vi "Sub_GBD_FileConvert.vi"(8 "error in (no error)":errorcluster, 10 "CSV":path caption="出力パス", 11 "GBD":path caption="ファイル") -> (0 "error out":errorcluster, 1 "EOF":bool)   [LabVIEW 2017]
panel:
  in  "Cancel Button":bool
  out "Slide":dbl(slide) scale=0.0..1.0
  in  "Param":cluster{"START":i32, "End":i32, "Delta":i32}={"START"=0, "End"=-1, "Delta"=1}
  # "ファイル変換中..."
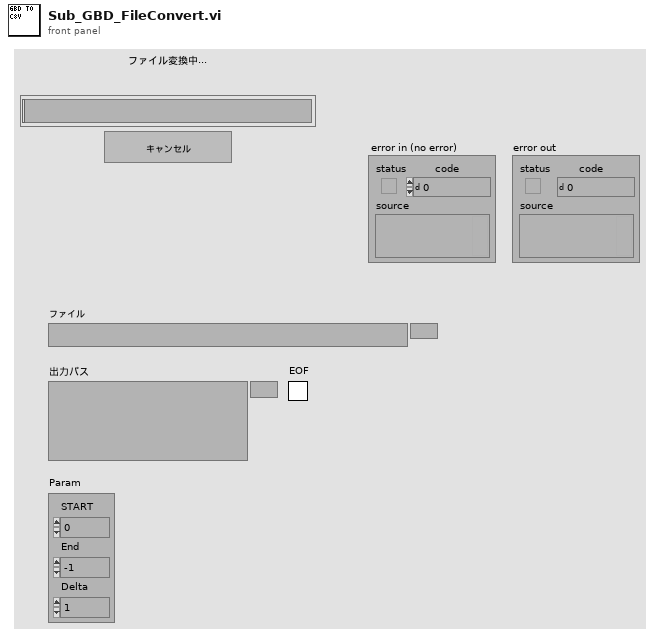
[diagram p1: front panel]
types:
  T1 = typedef "Amp_Param.ctl" = cluster{"File":refnum<file>[], "Idx":refnum<file>[], "dT":dbl, "Hd":i32, "Rd":i32, "Start":timestamp[], "Trig":timestamp[], "Stop":timestamp[], "FirstPos":timestamp[], "Count":i64[], "Color":u32[], "Label":string[], "INP":string[], "H":dbl[], "L":dbl[], "Fmt":string[], "Unit":string[], "SEL":i32[], "Byte":i32[], "Pos":i32[], "Bit":i32[], "Flg":i32[], "Gain":dbl[], "Offset":dbl[], "CH":i32[], "Opt":cluster{"Mode":i32, "TUNIT":enum16{"CELS", "FAHR"}}, "TYPE":enum16{"GBD", "CSV"}, "Comp":refnum<file>[], "Temp":i32[]}
  T2 = enum16{"open", "replace", "create", "open or create", "replace or create", "replace or create with confirmation"}
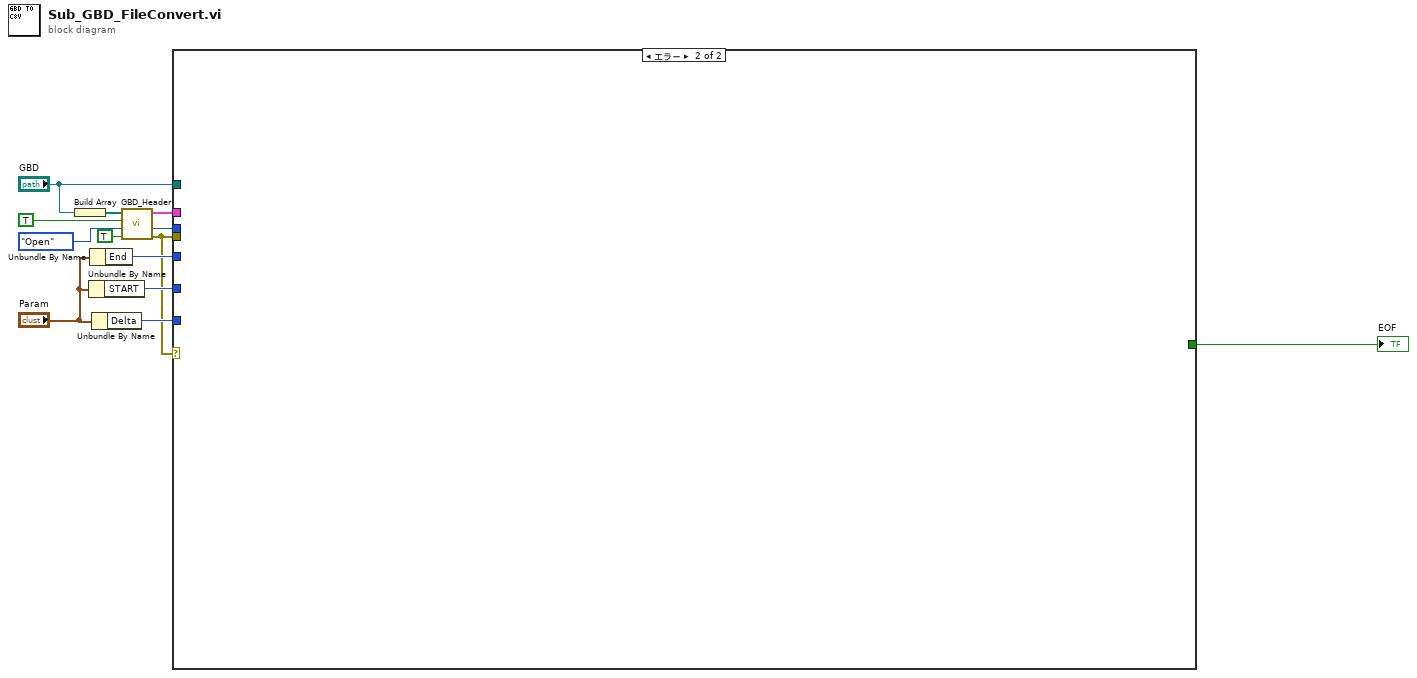
[diagram p0: block diagram]
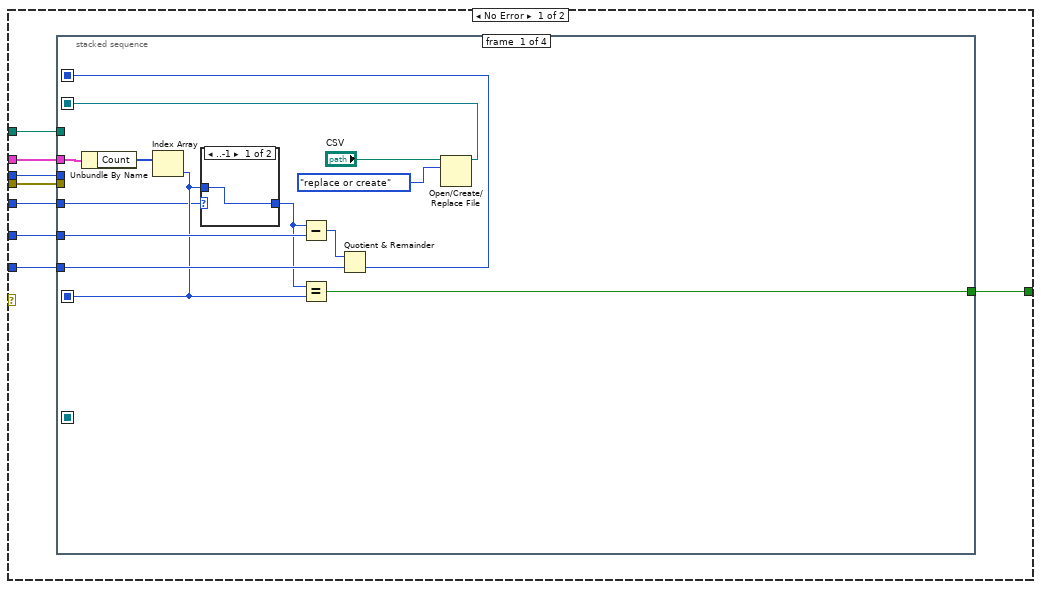
[diagram p2: hidden frame]
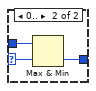
[diagram p3: hidden frame]
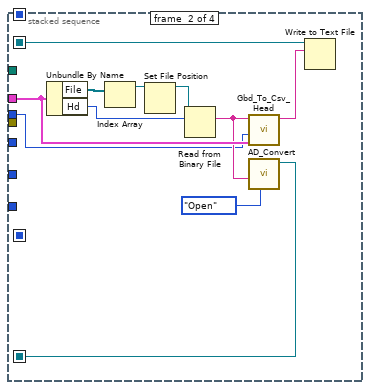
[diagram p4: hidden frame]
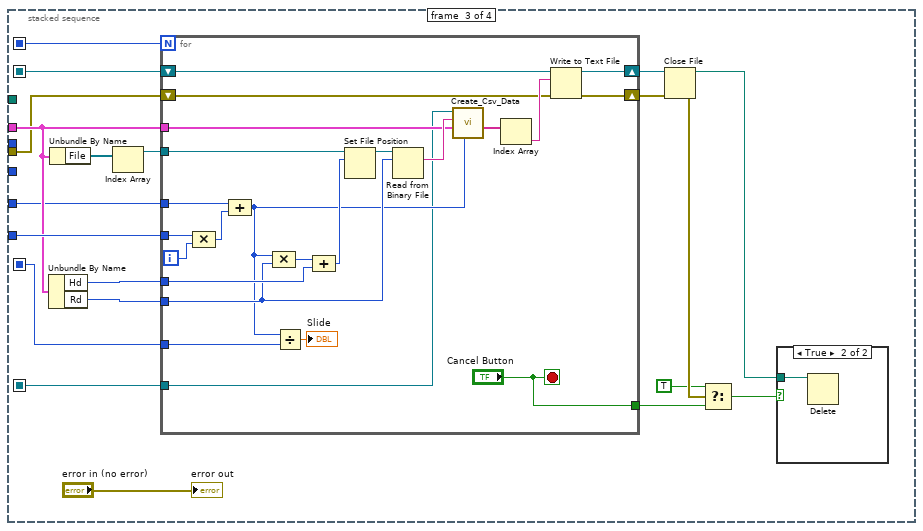
[diagram p5: hidden frame]
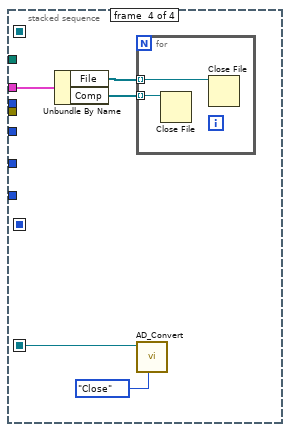
[diagram p7: hidden frame]
diagram:
  n1 = Build Array("GBD") -> (w3:path[])
  n2 = Unbundle By Name("Param") -> ("START"=w11:i32)
  n3 = Unbundle By Name("Param") -> ("End"=w12:i32)
  n4 = Unbundle By Name("Param") -> ("Delta"=w13:i32)
  n5 = call "GBD_Header.vi"("Save?"=TRUE, "Mode"=enum16{"Open", "Close", "Index"}."Open", "Cvt_Mode"=TRUE, "File[]"=w3) -> ("error out"=w1:errorcluster, "ActiveCH"=w2:i32, "Param"=w5:T1)  [unwired: 3 in, 2 out]
  n6 = case shown="エラー" w1 {
    tunnel: w13 -> [w21 _]
    tunnel: w12 -> [w20 _]
    tunnel: w11 -> [w19 _]
    tunnel: [w18 _] -> w9
    tunnel: "GBD" -> [w17 _]
    tunnel: w5 -> [w16 _]
    tunnel: w1 -> [w15 _]
    tunnel: w2 -> [w14 _]
    frame No Error {
      n7 = stacked-sequence {
        seq-local: [w33 _ _ _] -> [_ w45 w58 _]
        seq-local: [w28 _ _ _] -> [_ _ w64 _]
        seq-local: [w25 _ _ _] -> [_ _ w63 _]
        seq-local: [_ w40 _ _] -> [_ _ w55 w95]
        tunnel: w17 -> [_ _ _ _]
        tunnel: w19 -> [w31 _ w60 _]
        tunnel: w21 -> [w29 _ w65 _]
        tunnel: w20 -> [w24 _ _ _]
        tunnel: [w26 _ _ _] -> w18
        tunnel: w16 -> [w22 w43 w61 w98]
        tunnel: w15 -> [_ _ w54 _]
        tunnel: w14 -> [_ w39 _ _]
        frame #0 {
          n8 = Unbundle By Name(w22) -> ("Count"=w32:i64[])
          n9 = Index Array(array=w32) -> (element=w25:i64)  [unwired: 1 in]
          n10 = case shown="..-1" w24 {
            selector: w24 -> [_ w36]
            tunnel: [w35 w38] -> w27
            tunnel: w25 -> [w35 w37]
            frame ..-1 {
            }
            frame 0.. {
              n11 = Max & Min(x=w37, y=w36) -> (min(x,y)=w38:i64)  [unwired: 1 out]
            }
          }
          n12 = Subtract(x=w27, y=w31) -> (x-y=w30:i64)
          n13 = Equal?(x=w27, y=w25) -> (x = y?=w26:bool)
          n14 = Quotient & Remainder(x=w30, y=w29) -> (floor(x/y)=w28:i64)  [unwired: 1 out]
          n15 = Open/Create/Replace File(file path (use dialog)="CSV", operation (0:open)=T2."replace or create") -> (refnum out=w33:refnum<file>)  [unwired: 4 in, 2 out]
        }
        frame #1 {
          n16 = Unbundle By Name(w43) -> ("File"=w49:refnum<file>[], "Hd"=w46:i32)
          n17 = Index Array(array=w49) -> (element=w48:refnum<file>)  [unwired: 1 in]
          n18 = Set File Position(refnum=w48) -> (refnum out=w47:refnum<file>)  [unwired: 3 in, 1 out]
          n19 = Read from Binary File(10:w46, 11:w47) -> (2:w42:string)  [unwired: 4 in, 3 out]
          n20 = call "Gbd_To_Csv_Head.vi"("Param"=w43, "数値"=w39, "GBD"=w42) -> ("CSV"=w44:string)  [unwired: 8 in]
          n21 = call "AD_Convert.vi"("Mode"=enum16{"Open", "Convert", "Close"}."Open", "Header"=w42) -> ("Reference.Out"=w40:refnum<k24>)  [unwired: 7 in, 2 out]
          n22 = Write to Text File(file (use dialog)=w45, text=w44) -> ()  [unwired: 2 in, 3 out]
        }
        frame #2 {
          n23 = Unbundle By Name(w61) -> ("Hd"=w66:i32, "Rd"=w67:i32)
          n24 = Unbundle By Name(w61) -> ("File"=w69:refnum<file>[])
          n25 = Index Array(array=w69) -> (element=w68:refnum<file>)  [unwired: 1 in]
          n26 = for {
            N: w64 -> [_]
            tunnel: w68 -> [w93]
            tunnel: w67 -> [w87]
            tunnel: w66 -> [w90]
            tunnel: w60 -> [w83]
            tunnel: w65 -> [w85]
            tunnel: w63 -> [w81]
            tunnel: w61 -> [w78]
            tunnel: ["Cancel Button"] -> w52
            shift-right: [w76] -> w59
            shift-left: w58 -> [w75]
            tunnel: w55 -> [w72]
            shift-right: [w74] -> w56
            shift-left: w54 -> [w71]
            i -> [w84]
            stop <- "Cancel Button" stop-if-true
            n27 = Compound Arithmetic op=MULTIPLY(w85, w84) -> (w82:i32)
            n28 = Compound Arithmetic op=ADD(w83, w82) -> (w73:i32)
            n29 = Compound Arithmetic op=MULTIPLY(w73, w87) -> (w86:i32)
            n30 = Divide(x=w73, y=w81) -> (x/y=→"Slide":dbl)
            n31 = Compound Arithmetic op=ADD(w86, w90) -> (w92:i32)
            n32 = Set File Position(offset (in bytes) (0)=w92, refnum=w93) -> (refnum out=w91:refnum<file>)  [unwired: 2 in, 1 out]
            n33 = Read from Binary File(10:w87, 11:w91) -> (2:w89:string)  [unwired: 4 in, 3 out]
            n34 = call "Create_Csv_Data.vi"("N"=w73, "Head"=w78, "Bin"=w89, "Reference"=w72) -> ("CSV"=w80:string[])  [unwired: 5 in, 2 out]
            n35 = Index Array(array=w80) -> (element=w88:string)  [unwired: 1 in]
            n36 = Write to Text File(file (use dialog)=w75, text=w88, error in=w71) -> (refnum out=w76:refnum<file>, error out=w74:errorcluster)  [unwired: 1 in, 1 out]
          }
          n37 = Close File(refnum=w59, error in=w56) -> (path=w57:path, error out=w53:errorcluster)
          n38 = Select(t=TRUE, s=w53, f=w52) -> (s? t:f=w51:bool)
          n39 = case shown="TRUE" w51 {
            tunnel: w57 -> [_ w70]
            frame False {
            }
            frame True {
              n40 = Delete(path (use dialog)=w70) -> ()  [unwired: 4 in, 3 out]
            }
          }
          "error out" <- "error in (no error)"
        }
        frame #3 {
          n41 = Unbundle By Name(w98) -> ("File"=w97:refnum<file>[], "Comp"=w96:refnum<file>[])
          n42 = for {
            tunnel: w97 -> [w100] mode=indexing
            tunnel: w96 -> [w99] mode=indexing
            n43 = Close File(refnum=w99) -> ()  [unwired: 1 in, 2 out]
            n44 = Close File(refnum=w100) -> ()  [unwired: 1 in, 2 out]
          }
          n45 = call "AD_Convert.vi"("Mode"=enum16{"Open", "Convert", "Close"}."Close", "Reference.In"=w95) -> ()  [unwired: 7 in, 3 out]
        }
      }
    }
    frame Error {
    }
  }
  "EOF" <- w9
